vi "Update Autonomous Play Files.vi"() -> (6 "Application Directory":path, 8 "FileName\nFilepath\nArray":cluster{string, string}[](array[cluster]), 10 "Filepath Array":string[](array[string]), 15 "filename array":string[](array[string]))   [LabVIEW 2014]
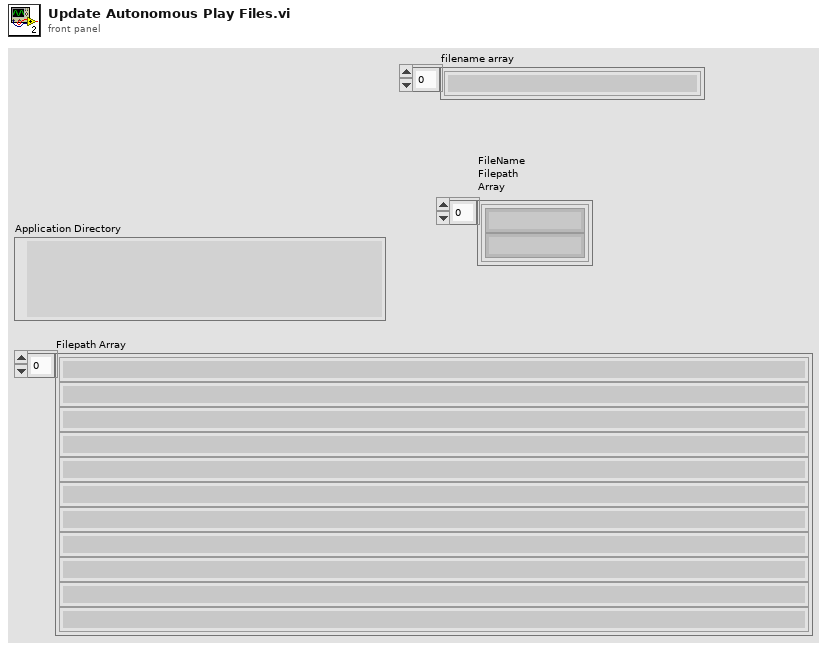
[diagram p1: front panel]
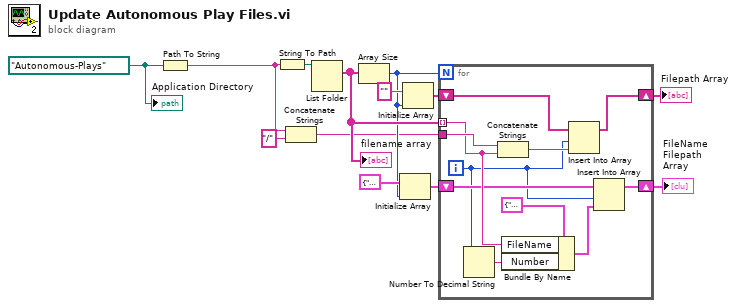
[diagram p0: block diagram]
diagram:
  w4 = path "/Autonomous-Plays" ("path")
  n1 = Path To String(path=w4) -> (string=w3:string)
  n2 = String To Path(string=w3) -> (path=w9:path)
  n3 = Concatenate Strings(w3, "/" ("string")) -> (w2:string)
  n4 = List Folder(path=w9) -> (filenames=w10:string[])  [unwired: 3 in, 3 out]
  "filename array" <- w10
  n5 = Array Size(array=w10) -> (size(s)=w6:i32)
  n6 = Initialize Array(cluster{string, string} {"", ""}, w6) -> (w8:cluster{string, string}[])
  n7 = Initialize Array("", w6) -> (w12:string[])
  n8 = for {
    N: w6 -> [_]
    tunnel: w10 -> [w21] mode=indexing
    tunnel: w2 -> [w24]
    shift-right: [w20] -> w13
    shift-left: w12 -> [w19]
    shift-right: [w16] -> w5
    shift-left: w8 -> [w18]
    i -> [w14]
    n9 = Number To Decimal String(number=w14) -> (decimal integer string=w15:string)  [unwired: 1 in]
    n10 = Concatenate Strings(w24, w21) -> (w22:string)
    n11 = Bundle By Name(cluster=cluster{"FileName":string, "Number":string} {"FileName"="", "Number"=""} ("input cluster"), "FileName"=w21, "Number"=w15) -> (w17:cluster{"FileName":string, "Number":string})
    n12 = Insert Into Array(array=w19, index=w14, new element=w22) -> (w20:string[])
    n13 = Insert Into Array(array=w18, index=w14, new element=w17) -> (w16:cluster{string, string}[])
  }
  "Filepath Array" <- w13
  "FileName\nFilepath\nArray" <- w5
  "Application Directory" <- w4
